vi "chrono.vi"() -> ()   [LabVIEW 2026]
panel:
  out "Client":string
  out "x-y":u32
  out "Numeric":i32
  in  "stop":bool
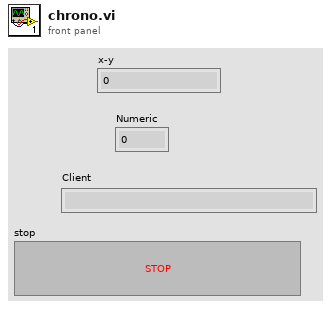
[diagram p1: front panel]
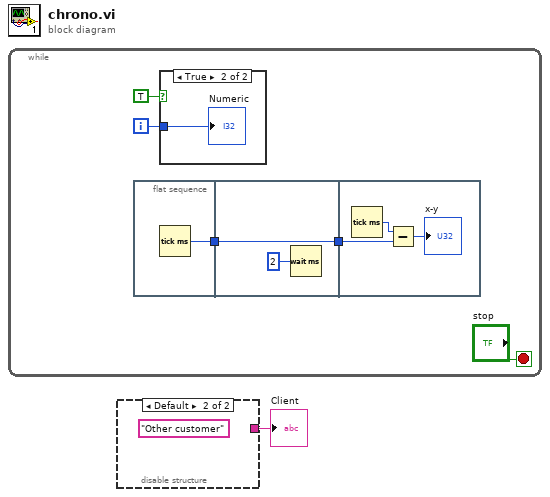
[diagram p0: block diagram]
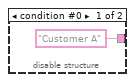
[diagram p3: hidden frame]
diagram:
  n1 = while {
    i -> [w5]
    stop <- "stop" stop-if-true
    n2 = flat-sequence {
      tunnel: [w8] -> w3
      tunnel: [w9] -> w4
      tunnel: w3 -> [w9]
      tunnel: w4 -> [w13]
      frame #0 {
        n3 = Tick Count (ms)() -> (millisecond timer value=w8:u32)
      }
      frame #1 {
        n4 = Wait (ms)(milliseconds to wait=u32 2) -> ()  [unwired: 1 out]
      }
      frame #2 {
        n5 = Tick Count (ms)() -> (millisecond timer value=w12:u32)
        n6 = Subtract(x=w12, y=w13) -> (x-y=→"x-y":u32)
      }
    }
    n7 = case shown="True" TRUE {
      tunnel: w5 -> [_ w7]
      frame False {
      }
      frame True {
        "Numeric" <- w7
      }
    }
  }
  n8 = disable-structure shown="Default" {
    disable-tunnel: ["Customer A" ("Client") _] -> w1
    frame condition #0 {
    }
    frame condition #1 (active) {
      (unwired) "Other customer" ("Client")
    }
  }
  "Client" <- w1
